vi "scrollbar_index.vi"(8 "error in (no error)":errorcluster, 9 "seek":i32, 10 "width_height":u32, 11 "data_available":i32) -> (0 "error out":errorcluster, 2 "length":i32=-1, 3 "index":i32=-1)   [LabVIEW 2015, in "lv-graph.lvlib"]
doc: "This VI will relegate scrollbar values with the data available and what's visible on the graph."
uses:
  lv-graph.lvlib
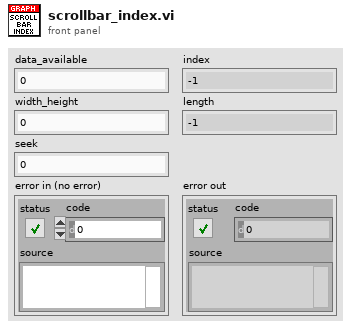
[diagram p1: front panel]
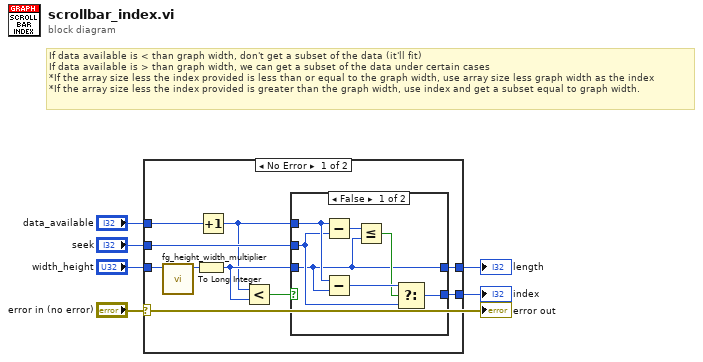
[diagram p0: block diagram]
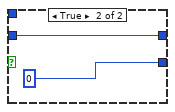
[diagram p2: hidden frame]
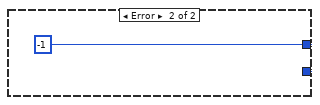
[diagram p3: hidden frame]
diagram:
  # "If data available is < than graph width, don't get a subset of the data (it'll fit)\nIf data available is > than graph width, we can get a subset of the data under certain cases\n*If the array size less the index provided is less than or equal to the graph width, use array size less graph width as the index\n*If the array size less the index provided is greater than the graph width, use index and get a subset equal to graph width."
  n1 = case shown="No Error" "error in (no error)" {
    tunnel: "seek" -> [w14 _]
    tunnel: "width_height" -> [w11 _]
    tunnel: [w10 w25] -> w4
    tunnel: [w9 w25] -> w3
    tunnel: "data_available" -> [w8 _]
    frame No Error {
      n2 = call "fg_height_width_multiplier.vi"("width_height in"=w11) -> ("width_height out"=w12:u32)  [unwired: 10 in]
      n3 = To Long Integer(number=w12) -> (32bit integer=w13:i32)
      n4 = Increment(x=w8) -> (x+1=w7:i32)
      n5 = Less?(x=w7, y=w13) -> (x < y?=w15:bool)
      n6 = case shown="False" w15 {
        tunnel: w7 -> [w21 _]
        tunnel: w13 -> [w16 w24]
        tunnel: w14 -> [w18 _]
        tunnel: [w17 0 ("Seek")] -> w10
        tunnel: [w16 w24] -> w9
        frame False {
          n7 = Subtract(x=w21, y=w18) -> (x-y=w22:i32)
          n8 = Subtract(x=w21, y=w16) -> (x-y=w20:i32)
          n9 = Less Or Equal?(x=w22, y=w16) -> (x <= y?=w19:bool)
          n10 = Select(t=w20, s=w19, f=w18) -> (s? t:f=w17:i32)
        }
        frame True {
        }
      }
    }
    frame Error {
      w25 = -1 ("Seek")
    }
  }
  "index" <- w4
  "length" <- w3
  "error out" <- "error in (no error)"
